vi "Validate Horizontal Settings.vi"(8 "error in (no error)":errorcluster, 11 "Oscilloscope in":refnum<class "Oscilloscope.lvclass">) -> (0 "error out":errorcluster, 3 "Oscilloscope out":refnum<class "Oscilloscope.lvclass">)   [LabVIEW 2019, in "Oscilloscope.lvlib" / "Oscilloscope.lvclass"]
uses:
  Oscilloscope.lvclass
  Oscilloscope.lvclass/Oscilloscope.ctl
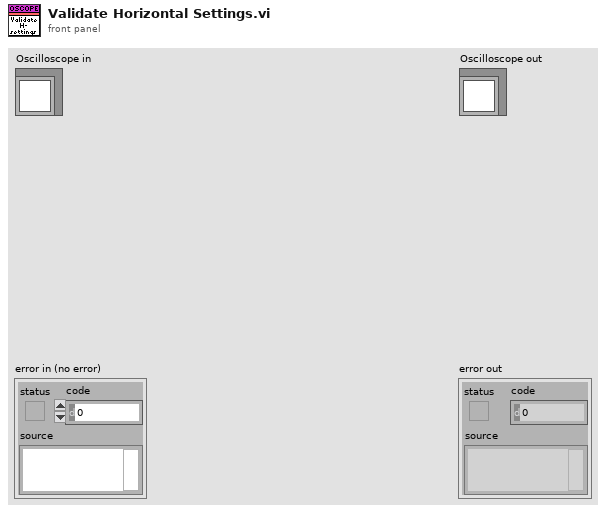
[diagram p1: front panel]
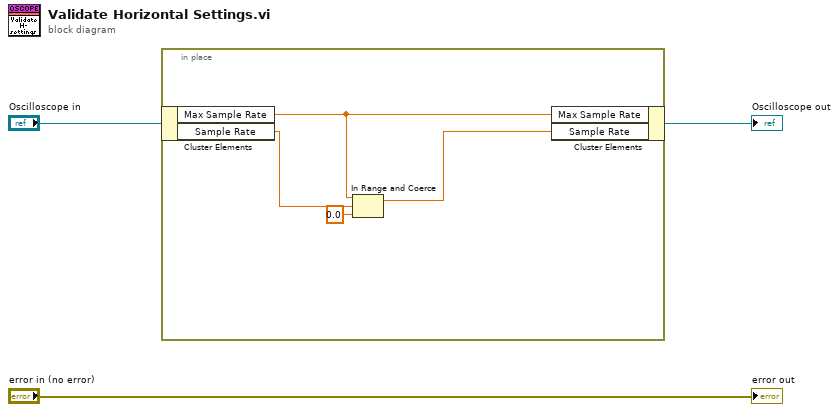
[diagram p0: block diagram]
diagram:
  n1 = in-place {
    n2 = in-place-cluster #1("Oscilloscope in") -> ("Max Sample Rate"=w5:dbl, "Sample Rate"=w7:dbl)
    n3 = In Range and Coerce(upper limit=w5, x=w7, lower limit=0.0) -> (coerced(x)=w6:dbl)  [unwired: 1 out]
    n4 = in-place-cluster #1("Max Sample Rate"=w5, "Sample Rate"=w6) -> (→"Oscilloscope out":refnum<class "Oscilloscope.lvclass">)
  }
  "error out" <- "error in (no error)"
